vi "Increment Write Address.vi"(8 "INC?":bool, 10 "Reset?":bool, 11 "rollover":u16) -> (0 "Input Valid":bool, 1 "roll over":bool, 3 "count":u16)   [LabVIEW 2012]
doc: "This counter counts from 0....Rollover and then returns to zero\ne.g., If rollover is 2, counter moves as 0,1,2,0,1,2.....\n\n<Latency> = 1 Tick from Reset"
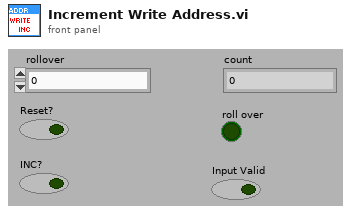
[diagram p1: front panel]
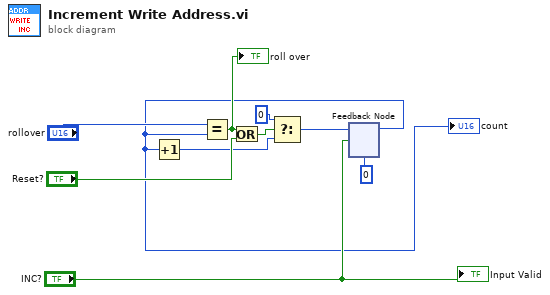
[diagram p0: block diagram]
diagram:
  n1 = feedback #1(u16 0) -> (w1:u16)
  "count" <- w1
  n2 = Increment(x=w1) -> (x+1=w2:u16)
  n3 = Equal?(x="rollover", y=w1) -> (x = y?=w8:bool)
  "roll over" <- w8
  n4 = Or(x=w8, y="Reset?") -> (x .or. y?=w7:bool)
  n5 = Select(t=u16 0, s=w7, f=w2) -> (s? t:f=w3:u16)
  n6 = feedback-in #1(w3, "INC?") -> ()
  "Input Valid" <- "INC?"
